vi "Init Image.vi"(8 "error in (no error)":errorcluster, 10 "Image Params":T1={"Mode"=enum."ROI", "Manual LUT"={"Minimum"=0.0, "Maximum"=0.0}, "BCG Values"={"Brightness"=128.0, "Contrast"=45.0, "Gamma"=1.0}, "Log?"=FALSE, "Auto?"=FALSE, "ROI"={"Global Rectangle"=[], "Contours"=[]}, "Image X"=0, "Image Y"=0, "HROI Pos"=0}, 11 "CameraPreview in":refnum<class "CameraPreview.lvclass">) -> (0 "error out":errorcluster, 3 "CameraPreview out":refnum<class "CameraPreview.lvclass">)   [LabVIEW 2023, in "CameraPreview.lvlib" / "CameraPreview.lvclass"]
uses:
  CameraPreview.lvclass
  CameraPreview.lvclass/CameraPreview.ctl
  Camera_Controller/Camera_Controller Messages/Image Init Done Msg/Image Init Done Msg.lvclass
  <vilib>/ActorFramework/Actor/Actor.lvclass
  typedefs/ImageProcessingParametersInPreview.ctl
  typedefs/typedefs.lvlib
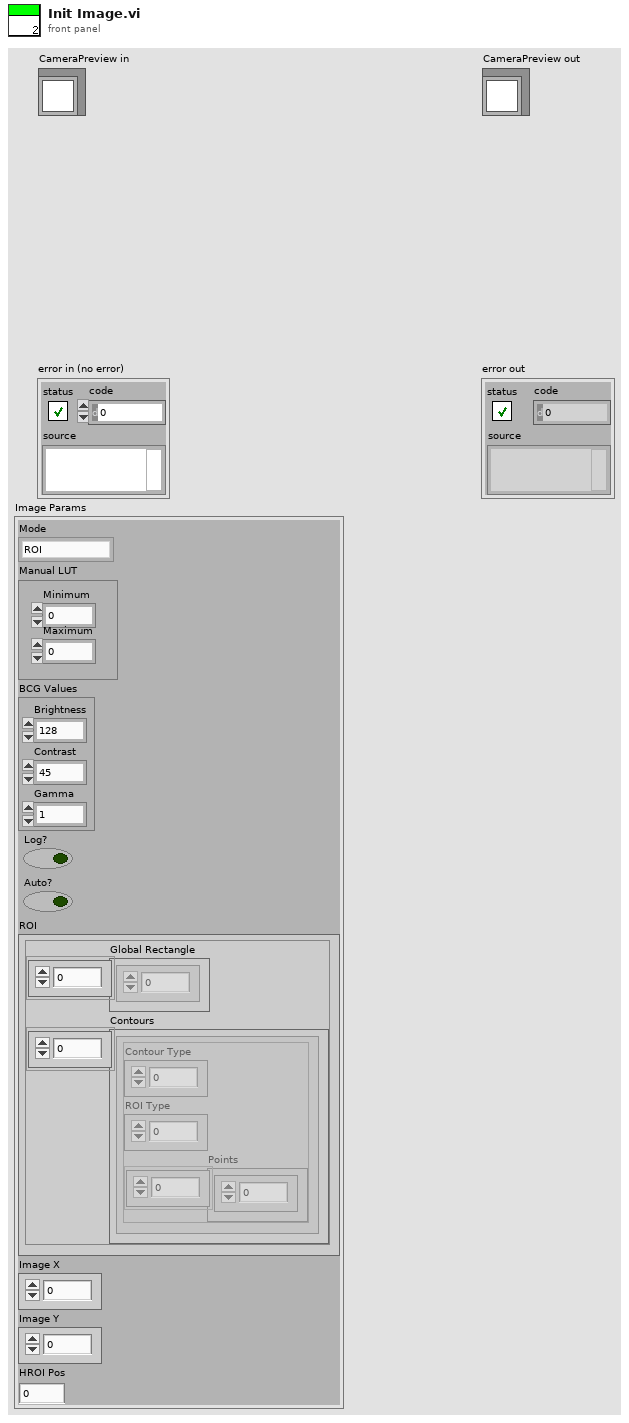
[diagram p1: front panel]
types:
  T1 = typedef "typedefs.lvlib/ImageProcessingParametersInPreview.ctl" = cluster{"Mode":enum16{"ROI", "Image"}, "Manual LUT":cluster{"Minimum":dbl, "Maximum":dbl}, "BCG Values":cluster{"Brightness":sgl, "Contrast":sgl, "Gamma":sgl}, "Log?":bool, "Auto?":bool, "ROI":cluster{"Global Rectangle":i32[], "Contours":cluster{"Contour Type":u32, "ROI Type":u32, "Points":i32[]}[]}, "Image X":i32, "Image Y":i32, "HROI Pos":u16}
  T2 = typedef "Image Type" = u32
  T3 = typedef "IMAQ Image.ctl" = refnum<image>
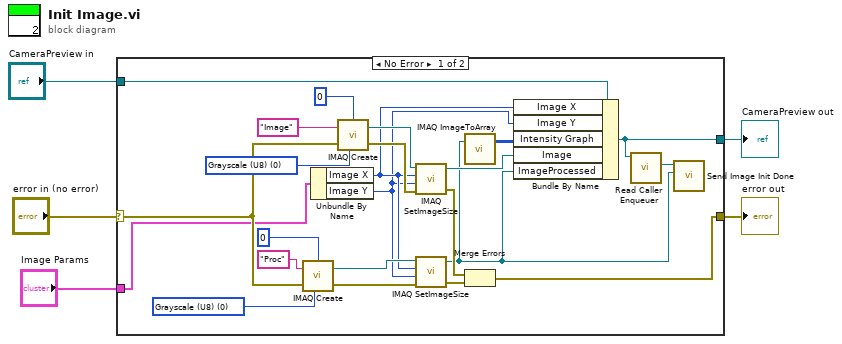
[diagram p0: block diagram]
diagram:
  n1 = case shown="No Error" "error in (no error)" {
    selector: "error in (no error)" -> [w11 w30]
    tunnel: [w17 w30] -> w4
    tunnel: [w8 w29] -> w2
    tunnel: "CameraPreview in" -> [w16 w29]
    tunnel: "Image Params" -> [w10 _]
    frame No Error {
      w12 = T2 0 items=["Grayscale (U8)", "Grayscale (I16)", "Grayscale (SGL)", "Complex (CSG)", "RGB (U32)", "HSL (U32)", "RGB (U64)", "Grayscale (U16)"] ("Image Type")
      w19 = T2 0 items=["Grayscale (U8)", "Grayscale (I16)", "Grayscale (SGL)", "Complex (CSG)", "RGB (U32)", "HSL (U32)", "RGB (U64)", "Grayscale (U16)"] ("Image Type")
      n2 = call "IMAQ Create"("Border Size"=0, "Image Name"="Proc", "Image Type"=w12, "error in (no error)"=w11) -> ("New Image"=w27:T3, "error out"=w22:errorcluster)  [unwired: 1 in]
      n3 = Unbundle By Name(w10) -> ("Image X"=w15:i32, "Image Y"=w14:i32)
      n4 = call "IMAQ Create"("Border Size"=0, "Image Name"="Image", "Image Type"=w19, "error in (no error)"=w11) -> ("New Image"=w21:T3, "error out"=w24:errorcluster)  [unwired: 1 in]
      n5 = call "IMAQ SetImageSize"("error in (no error)"=w24, "Y Resolution"=w14, "X Resolution"=w15, "Image"=w21) -> ("error out"=w25:errorcluster, "Image Out"=w26:T3)  [unwired: 1 in]
      n6 = call "IMAQ SetImageSize"("error in (no error)"=w22, "Y Resolution"=w14, "X Resolution"=w15, "Image"=w27) -> ("error out"=w23:errorcluster, "Image Out"=w6:T3)  [unwired: 1 in]
      n7 = call "IMAQ ImageToArray"("Image"=w6) -> ("Image Pixels (U8)"=w7:u8[][])  [unwired: 3 in, 4 out]
      n8 = Merge Errors(w25, w23) -> (w17:errorcluster)
      n9 = Bundle By Name(cluster=w16, "Image X"=w15, "Image Y"=w14, "Intensity Graph"=w7, "Image"=w26, "ImageProcessed"=w6) -> (w8:refnum<class "CameraPreview.lvclass">)
      n10 = call <vilib>:"Read Caller Enqueuer.vi"("Actor"=w8) -> ("Caller Enqueuer"=w9:refnum<class "Message Enqueuer.lvclass">)  [unwired: 10 in]
      n11 = call "Send Image Init Done.vi"("Processed Image"=w6, "Message Enqueuer"=w9) -> ()  [unwired: 8 in, 2 out]
    }
    frame Error {
    }
  }
  "error out" <- w4
  "CameraPreview out" <- w2
